vi "toml_lock_acquire.vi"(8 "error in (no error)":errorcluster, 11 "path in":path) -> (0 "error out":errorcluster, 1 "resolved path":path, 3 "lock":refnum<queue>)   [LabVIEW 2017]
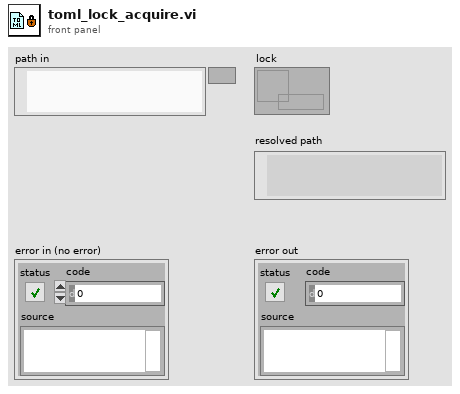
[diagram p1: front panel]
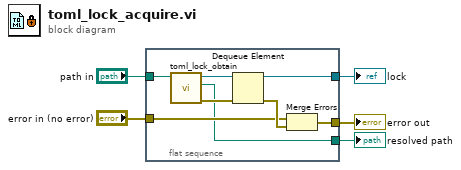
[diagram p0: block diagram]
diagram:
  n1 = flat-sequence {
    tunnel: "path in" -> [w7]
    tunnel: [w13] -> w4
    tunnel: [w11] -> w3
    tunnel: "error in (no error)" -> [w10]
    tunnel: [w6] -> w1
    frame #0 {
      n2 = call "toml_lock_obtain.vi"("path in"=w7) -> ("error out"=w9:errorcluster, "resolved path"=w6:path, "lock"=w8:refnum<queue>)  [unwired: 7 in, 1 out]
      n3 = Dequeue Element(queue=w8, error in (no error)=w9) -> (queue out=w13:refnum<queue>, error out=w12:errorcluster)  [unwired: 1 in, 2 out]
      n4 = Merge Errors(w10, w12) -> (w11:errorcluster)
    }
  }
  "lock" <- w4
  "error out" <- w3
  "resolved path" <- w1
